vi "test_10.vi"() -> ()   [LabVIEW 2016]
panel:
  in  "Boolean":bool
  in  "确定按钮":bool
  in  "VCI_INIT_CONFIG":T1={"AccCode"=0, "AccMask"=4294967295, "Reserved"=0, "Filter"=0, "Timing0"=0, "Timing1"=28, "Mode"=0} {"AccCode" format="%x"; "AccMask" format="%x"; "Reserved" format="%x"; "Timing1" format="%x"}
  out "InitCAN_Success":i32
  out "CloseDevice_Success":i32
  in  "VCI_CAN_OBJ":T2={"ID"=255, "TimeStamp"=0, "TimeFlag"=0, "SendType"=0, "RemoteFlag"=0, "ExternFlag"=0, "DataLen"=8, "Data"=1, 1, 1, 1, 1, 1, 1, 1, "Reserved"=0, 0, 0} {"ID" format="%x"}
  out "SendNUM":i32=1
  out "VCI_CAN_OBJ":T3={"ID"=255, "TimeStamp"=0, "TimeFlag"=0, "SendType"=0, "RemoteFlag"=0, "ExternFlag"=0, "DataLen"=8, "Data"=1, 1, 1, 1, 1, 1, 1, 1, "Reserved"=0, 0, 0}
  out "recNUM":u32=1
  in  "停止":bool
  out "StartCAN_Success":i32
  out "OpenDevice":i32
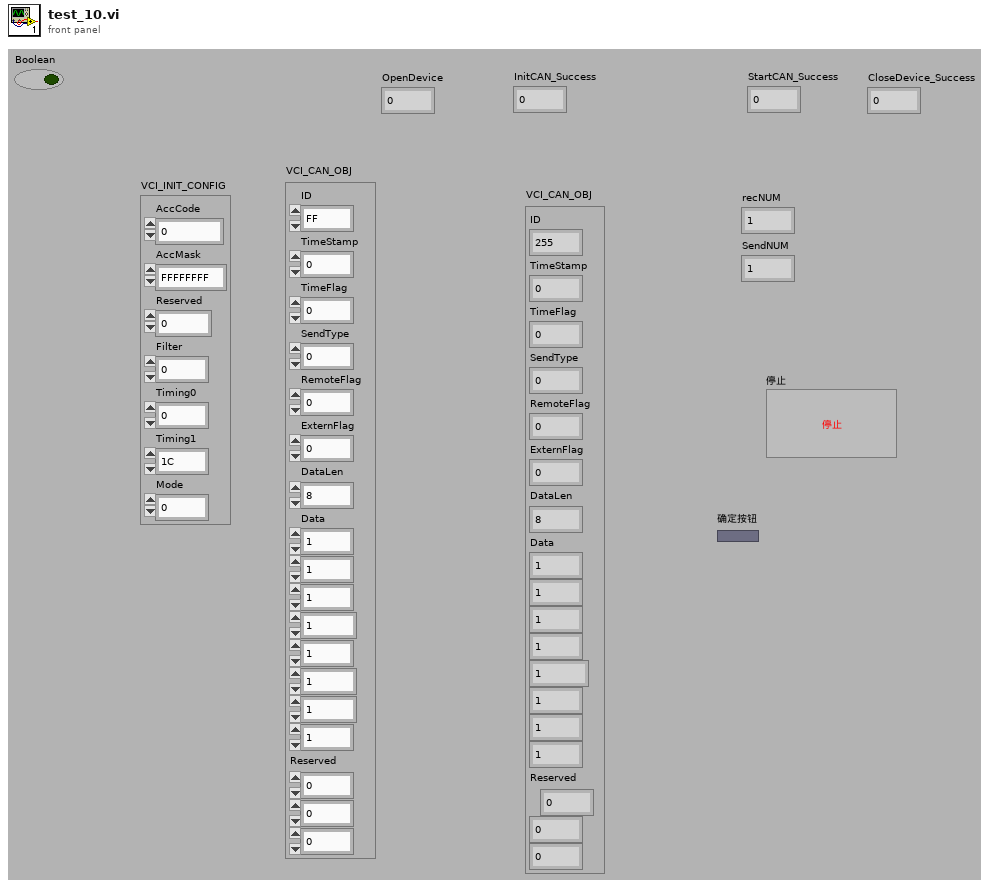
[diagram p1: front panel]
types:
  T1 = cluster{"AccCode":u32, "AccMask":u32, "Reserved":u32, "Filter":u8, "Timing0":u8, "Timing1":u8, "Mode":u8}
  T2 = cluster{"ID":u32, "TimeStamp":u32, "TimeFlag":u8, "SendType":u8, "RemoteFlag":u8, "ExternFlag":u8, "DataLen":u8, "Data":u8, u8, u8, u8, u8, u8, u8, u8, "Reserved":u8, u8, u8}
  T3 = cluster{"ID":u32, "TimeStamp":u32, "TimeFlag":i8, "SendType":i8, "RemoteFlag":i8, "ExternFlag":i8, "DataLen":i8, "Data":u8, u8, u8, u8, u8, u8, u8, u8, "Reserved":u8, u8, u8}
  T4 = cluster{"ID":u32, "TimeStamp":u32, "TimeFlag":u8, "SendType":i8, "RemoteFlag":u8, "ExternFlag":u8, "DataLen":u8, "Data0":u8, "Data1":u8, "Data2":u8, "Data3":u8, "Data4":u8, "Data5":u8, "Data6":u8, "Data7":u8, "Reserved":u8, u8, u8}
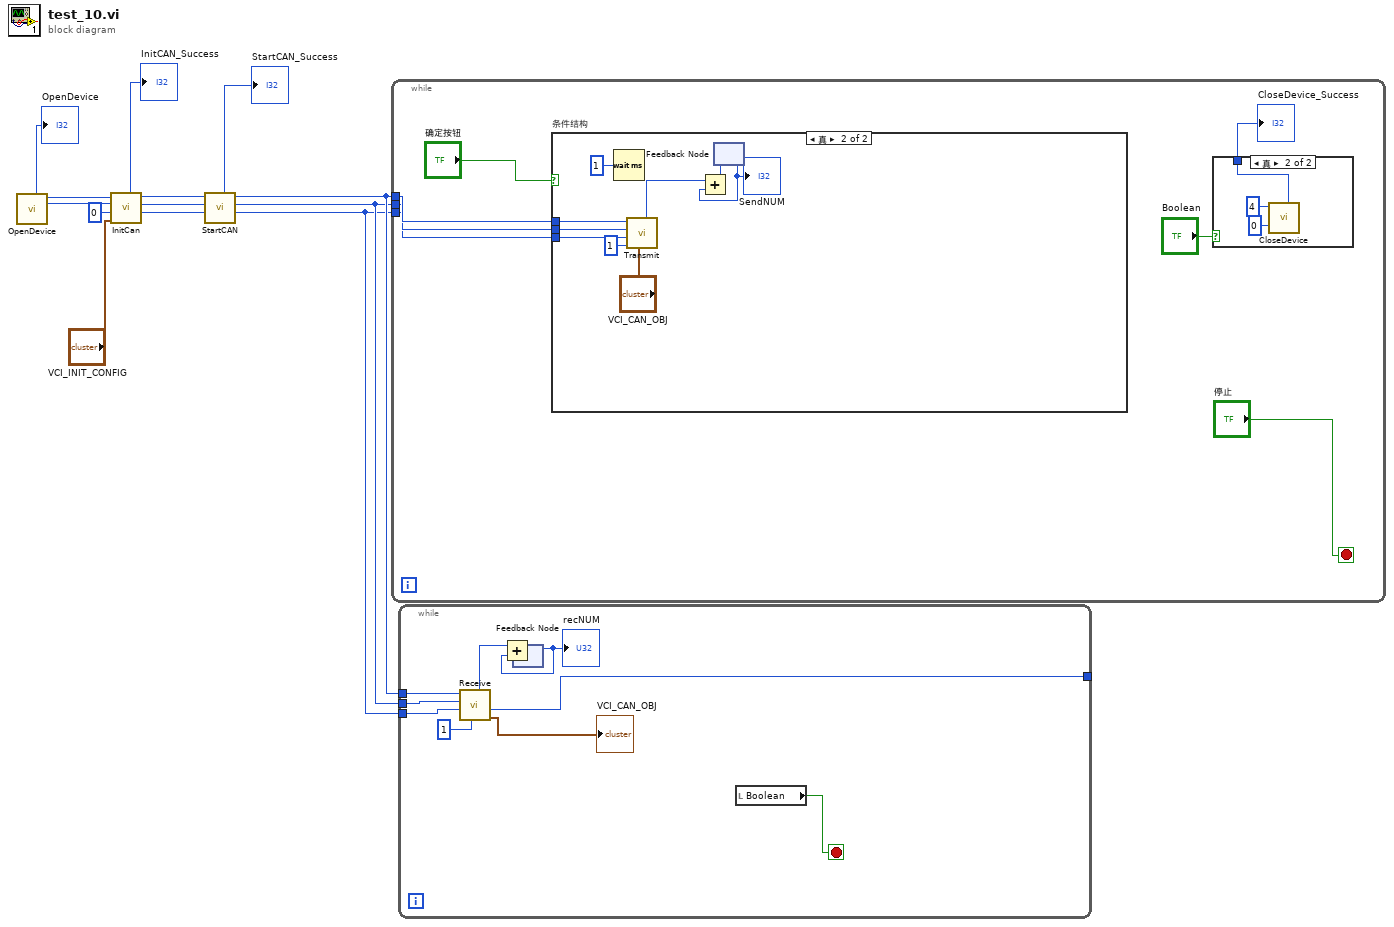
[diagram p0: block diagram]
diagram:
  n1 = call "OpenDevice.vi"() -> ("DevIndex"=w12:u32, "DevType"=w13:u32, "OpenDevice"=→"OpenDevice":i32)  [unwired: 9 out]
  n2 = call "InitCan.vi"("VCI_INIT_CONFIG"="VCI_INIT_CONFIG", "CanIndex_IN"=u32 0, "DevIndex_IN"=w12, "DevType_IN"=w13) -> ("CanIndex_OUT"=w3:u32, "DevIndex_OUT"=w4:u32, "DevType_OUT"=w2:u32, "InitCAN_Success?"=→"InitCAN_Success":u32)  [unwired: 4 out]
  n3 = call "StartCAN.vi"("CANIndex"=w3, "DevIndex"=w4, "DevType"=w2) -> ("CANIndex 2"=w6:u32, "DevIndex 2"=w7:u32, "DevType 2"=w8:u32, "StartCAN_Success?"=→"StartCAN_Success":u32)  [unwired: 5 out]
  n4 = while {
    tunnel: w8 -> [w20]
    tunnel: w7 -> [w19]
    tunnel: w6 -> [w18]
    stop <- "停止" stop-if-true
    n5 = case "条件结构" shown="真" "确定按钮" {
      tunnel: w20 -> [_ w32]
      tunnel: w19 -> [_ w31]
      tunnel: w18 -> [_ w30]
      frame False {
      }
      frame True {
        n6 = Wait (ms)(milliseconds to wait=u32 1 ("等待时间（毫秒）")) -> ()  [unwired: 1 out]
        n7 = call "Transmit.vi"("VCI_CAN_OBJ"="VCI_CAN_OBJ", "Len"=u32 1, "CANIndex"=w30, "DevIndex"=w31, "DevType"=w32) -> ("sendNUM"=w27:i32)  [unwired: 6 out]
        n8 = feedback #1() -> (w25:i32)  [unwired: 1 in]
        "SendNUM" <- w25
        n9 = Add(x=w27, y=w25) -> (x+y=w26:i32)
        n10 = feedback-in #1(w26) -> ()
      }
    }
    n11 = case shown="真" "Boolean" {
      tunnel: [_ w23] -> w16
      frame False {
      }
      frame True {
        n12 = call "CloseDevice.vi"("DevIndex"=u32 0, "DevType"=u32 4) -> ("CloseDevice_Success?"=w23:u32)  [unwired: 9 out]
      }
    }
    "CloseDevice_Success" <- w16
  }
  n13 = while {
    tunnel: w8 -> [w42]
    tunnel: w7 -> [w41]
    tunnel: w6 -> [w40]
    tunnel: [w38] -> _
    stop <- w33 stop-if-true
    n14 = call "Receive.vi"("Len"=u32 1, "CANIndex"=w40, "DevIndex"=w41, "DevType"=w42) -> ("VCI_CAN_OBJ"=→"VCI_CAN_OBJ":T4, "CANIndex 2"=w38:u32, "RecNUM"=w37:i32)  [unwired: 1 in, 4 out]
    n15 = feedback #2() -> (w35:i32)  [unwired: 1 in]
    "recNUM" <- w35
    n16 = Add(x=w37, y=w35) -> (x+y=w36:i32)
    n17 = feedback-in #2(w36) -> ()
    n18 = local read "Boolean"() -> (w33:bool)
  }
